vi "Transaction.vi"(8 "Error In":errorcluster, 9 "Bytes to read (100)":u32=100, 10 "Command":string, 11 "VISA resource name":refnum<visa-resource-name>) -> (0 "Error Out":errorcluster, 2 "Response":string, 3 "dup VISA resource name":refnum<visa-resource-name>)   [LabVIEW 2011, in "MGC647C.lvlib"]
doc: "This VI handles the low level communication with the device.\n\nIt adds/removes formatting characters (CR/LF) and parses error information into the error cluster."
uses:
  <instrlib>/MGC647C/MGC647C.lvlib
  <userlib>/FGV_Utilities/HGF_FGV_File/Action Text File.ctl
  <userlib>/FGV_Utilities/HGF_FGV_File/HGF_FGV_File.lvlib
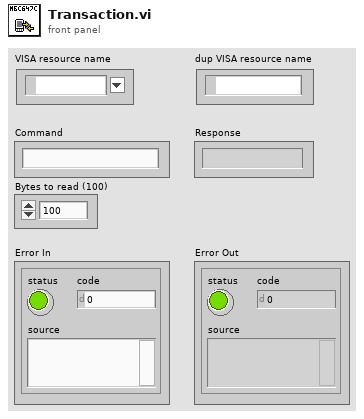
[diagram p1: front panel]
types:
  T1 = typedef "Semaphore RefNum" = refnum<k1>
  T2 = typedef "HGF_FGV_File.lvlib/Action Text File.ctl" = enum16{"open file", "read lines", "read characters", "write", "flush", "close file", ""}
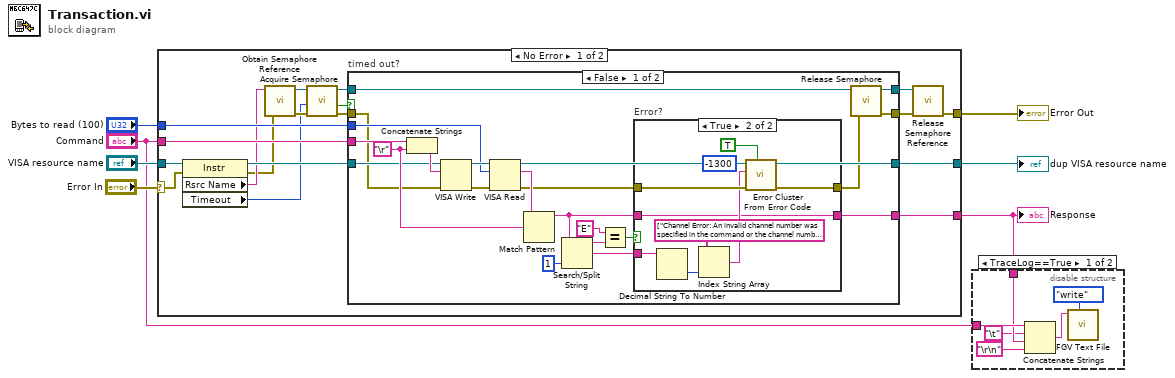
[diagram p0: block diagram]
diagram:
  n1 = case shown="No Error" "Error In" {
    selector: "Error In" -> [w19 w62]
    tunnel: "VISA resource name" -> [w21 w63]
    tunnel: [w25 w63] -> w6
    tunnel: "Bytes to read (100)" -> [w24 _]
    tunnel: "Command" -> [w23 _]
    tunnel: [w9 w62] -> w4
    tunnel: [w22 _] -> w1
    frame No Error {
      n2 = property class="Instr"(reference=w21, error in=w19) -> (reference out=w20:refnum<visa-resource-name>, error out=w17:errorcluster, "Rsrc Name"=w18:string, "Timeout"=w14:u32)
      n3 = call <vilib>:"Obtain Semaphore Reference.vi"("error in (no error)"=w17, "name (unnamed)"=w18) -> ("error out"=w16:errorcluster, "semaphore"=w15:T1)  [unwired: 3 in, 1 out]
      n4 = call <vilib>:"Acquire Semaphore.vi"("error in (no error)"=w16, "ms timeout (-1)"=w14, "semaphore"=w15) -> ("error out"=w11:errorcluster, "timed out"=w13:bool, "semaphore out"=w12:T1)  [unwired: 2 in]
      n5 = case "timed out?" shown="False" w13 {
        tunnel: [w45 w61] -> w25
        tunnel: w24 -> [w44 _]
        tunnel: w23 -> [w43 _]
        tunnel: [w28 w60] -> w8
        tunnel: [w32 _] -> w22
        tunnel: w20 -> [w31 w61]
        tunnel: w12 -> [w29 w59]
        tunnel: w11 -> [w30 w60]
        tunnel: [w26 w59] -> w10
        frame False {
          w41 = "\r"
          n6 = Concatenate Strings(w43, w41) -> (w42:string)
          n7 = VISA Write(VISA resource name=w31, write buffer=w42, error in (no error)=w30) -> (VISA resource name out=w46:refnum<visa-resource-name>, error out=w47:errorcluster)  [unwired: 1 out]
          n8 = VISA Read(VISA resource name=w46, byte count=w44, error in (no error)=w47) -> (VISA resource name out=w45:refnum<visa-resource-name>, read buffer=w40:string, error out=w37:errorcluster)  [unwired: 1 out]
          n9 = Match Pattern(string=w40, regular expression=w41) -> (before substring=w33:string)  [unwired: 1 in, 3 out]
          n10 = Search/Split String(string=w33, offset (0)=1 ("length (rest)")) -> (substring before match=w35:string, match + rest of string=w34:string)  [unwired: 1 in, 1 out]
          n11 = Equal?(x="E" ("regular expression"), y=w35) -> (x = y?=w38:bool)
          n12 = case "Error?" shown="True" w38 {
            tunnel: w37 -> [w49 w58]
            tunnel: [w49 w57] -> w27
            tunnel: w34 -> [_ w55]
            tunnel: [w48 w51] -> w32
            tunnel: w33 -> [w48 w51]
            frame False {
            }
            frame True {
              n13 = Decimal String To Number(string=w55) -> (number=w53:i32)  [unwired: 2 in, 1 out]
              n14 = Index String Array(1:w53, 2:string[] ["Channel Error: An invalid channel number was specified in the command or the channel number is missing.", "Unknown command: A command has been transmitted which is unkown to the 647C.", "Syntax error: Only one character has been sent instead of the expected two byte command", "Invalid expression: The command paramter does not have decimal form, or invalid characters were found in the paramter (e.g. 100.3: the decimal point is an invalid character).", "Invalid value: The transmitted parameter is outside the paramter range (e.g. 1299 is outside the range of a set point).", "Auto zero error: There was a trial to set the  zero offset of an active channel. Before setting the zero offset, either the channel (OF #) or the gas (OF 0) has to be switched off."]) -> (0:w52:string)  [unwired: 1 in]
              n15 = call <vilib>:"Error Cluster From Error Code.vi"("show call chain? (False)"=TRUE, "error in (no error)"=w58, "error message (\"\")"=w52, "error code (0)"=-1300) -> ("error out"=w57:errorcluster)  [unwired: 5 in]
            }
          }
          n16 = call <vilib>:"Release Semaphore.vi"("error in (no error)"=w27, "semaphore"=w29) -> ("error out"=w28:errorcluster, "semaphore out"=w26:T1)  [unwired: 4 in]
        }
        frame True {
        }
      }
      n17 = call <vilib>:"Release Semaphore Reference.vi"("error in (no error)"=w8, "semaphore"=w10) -> ("error out"=w9:errorcluster)  [unwired: 8 in, 1 out]
    }
    frame Error {
    }
  }
  "dup VISA resource name" <- w6
  "Error Out" <- w4
  "Response" <- w1
  n18 = disable-structure shown="TraceLog==True" {
    disable-tunnel: "Command" -> [w68 _]
    disable-tunnel: w1 -> [w67 _]
    frame condition #0 (active) {
      n19 = Concatenate Strings(w68, "\t", w67, "\r\n") -> (w69:string)
      n20 = call <userlib>:"FGV Text File.vi"("Action"=Action_Text_File."write", "Text in"=w69) -> ()  [unwired: 7 in, 3 out]
    }
    frame condition #1 {
    }
  }
